vi "Collect.vi"(8 "error in (no error)":errorcluster, 11 "Collectable in":refnum<class "Collectable.lvclass">) -> (0 "error out":errorcluster, 2 "Metrics":refnum<data-value>[](array[refnum]), 3 "Collectable out":refnum<class "Collectable.lvclass">)   [LabVIEW 2020, in "Collector.lvlib" / "Collectable.lvclass"]
uses:
  Collectable.lvclass
  metrics/metric/Metric.lvclass
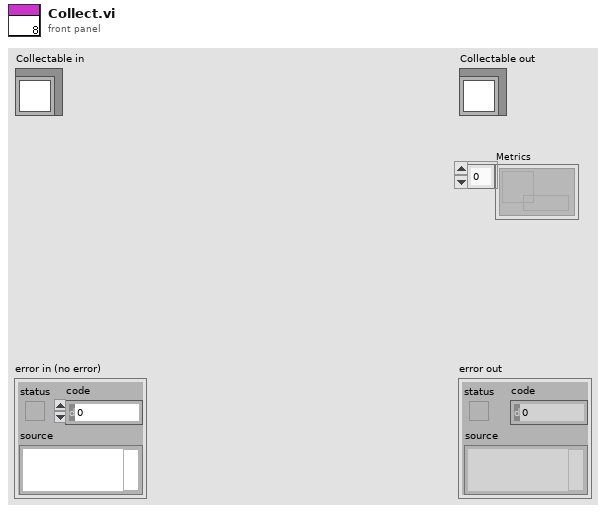
[diagram p1: front panel]
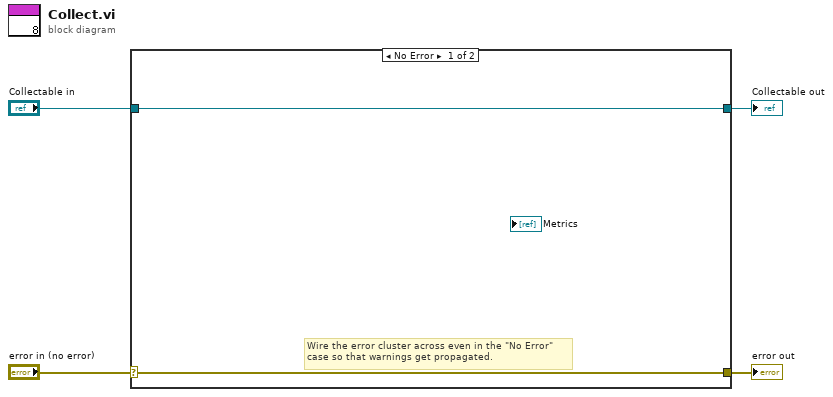
[diagram p0: block diagram]
diagram:
  n1 = case shown="No Error" "error in (no error)" {
    selector: "error in (no error)" -> [w5 w8]
    tunnel: [w5 w8] -> w3
    tunnel: [w6 w7] -> w1
    tunnel: "Collectable in" -> [w6 w7]
    frame No Error {
      # "Wire the error cluster across even in the \"No Error\"\ncase so that warnings get propagated."
    }
    frame Error {
    }
  }
  "error out" <- w3
  "Collectable out" <- w1
